vi "Receive Message.vi"(6 "priority":i32, 10 "Graph in":refnum<class "Graph.lvclass">, 11 "Message in":refnum<class "Message.lvclass">) -> (0 "error out":errorcluster, 2 "Actor out":refnum<class "Actor.lvclass">)   [LabVIEW 2020, in "Graph.lvlib" / "Graph.lvclass"]
doc: "This implementation filters for Data Msgs. If a Data Msg is recieved the contained data is forwarded to the UI of the Actor Core."
uses:
  Graph.lvclass
  PPL/HDH.Actor Framework.Core.Actor.lvlibp/1abvi3w/vi.lib/ActorFramework/Message/Message.lvclass
  PPL/HDH.Actor Framework.Core.Actor.lvlibp/1abvi3w/vi.lib/ActorFramework/Actor/Actor.lvclass
  C:/Current projects/WS/PPL/HDH.Actor Framework.Core.Actor.lvlibp/1abvi3w/vi.lib/ActorFramework/Actor/Actor.lvclass
  PPL/HDH.Actor Framework.Core.Publisher.lvlibp/Messages/Data Msg/Data Msg.lvclass
  Graph.lvclass/Graph.ctl
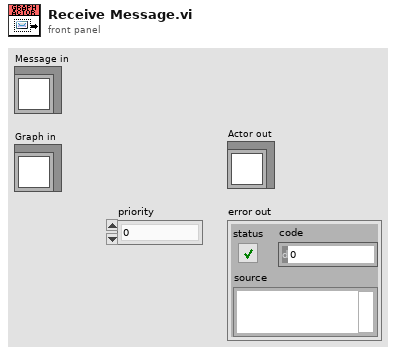
[diagram p1: front panel]
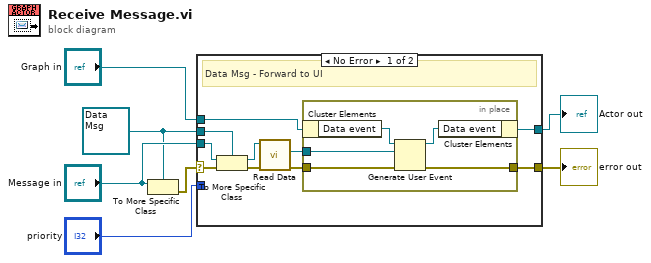
[diagram p0: block diagram]
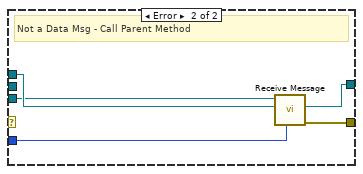
[diagram p2: hidden frame]
diagram:
  w2 = refnum<class "Data Msg.lvclass"> refnum ("HDH.Actor Framework.Core.Publisher.lvlibp:Data Msg.lvclass")
  n1 = To More Specific Class(target class=w2, reference="Message in") -> (error out=w3:errorcluster)  [unwired: 1 in, 1 out]
  n2 = case shown="No Error" w3 {
    selector: w3 -> [w17 _]
    tunnel: [w8 w27] -> w7
    tunnel: [w11 w26] -> w1
    tunnel: "priority" -> [_ w25]
    tunnel: "Graph in" -> [w12 w24]
    tunnel: "Message in" -> [w16 w23]
    tunnel: w2 -> [w15 _]
    frame No Error {
      # "Data Msg - Forward to UI"
      n3 = To More Specific Class(target class=w15, reference=w16, error in=w17) -> (specific class reference=w14:refnum<class "Data Msg.lvclass">, error out=w13:errorcluster)
      n4 = call "Read Data.vi"("error in (no error)"=w13, "Data Msg in"=w14) -> ("error out"=w9:errorcluster, "Data"=w10:refnum<class "Data.lvclass">)  [unwired: 7 in, 1 out]
      n5 = in-place {
        in-place-border: w10 -> [w20]
        in-place-border: w9 -> [w19]
        in-place-border: [w18] -> w8
        n6 = in-place-cluster #1(w12) -> ("Data event"=w22:refnum<user-event>)
        n7 = Generate User Event(user event=w22, event data cluster=w20, error in=w19) -> (user event out=w21:refnum<user-event>, error out=w18:errorcluster)  [unwired: 1 in]
        n8 = in-place-cluster #1("Data event"=w21) -> (w11:refnum<class "Graph.lvclass">)
      }
    }
    frame Error {
      # "Not a Data Msg - Call Parent Method"
      n9 = call-parent "Receive Message.vi"("priority"=w25, "Actor in"=w24, "Message in"=w23) -> ("error out"=w27:errorcluster, "Actor out"=w26:refnum<class "Actor.lvclass">)  [unwired: 7 in]
    }
  }
  "error out" <- w7
  "Actor out" <- w1
